vi "TicTacToe_pvp.vi"() -> ()   [LabVIEW 2020]
panel:
  in  "Turn 2":bool
  out "Human Win":dbl
  in  "Show XO plate":bool
  out "Computer Win":dbl
  out "Tie":bool
  out "No one Won":bool
  out "Game Over":bool
  out "Computer Won":bool
  out "Human Won":bool
  out "Turn":string
  out "XO array":string[][](array[string])
  in  "START GAME":bool
  in  "Boolean 9":bool
  in  "Boolean 8":bool
  in  "Boolean 7":bool
  in  "Boolean 6":bool
  in  "Boolean 5":bool
  in  "Boolean 4":bool
  in  "Boolean 3":bool
  in  "Boolean 2":bool
  in  "Boolean":bool
  in  "STOP GAME":bool
  in  "Turn":bool
  # "XO GAME"
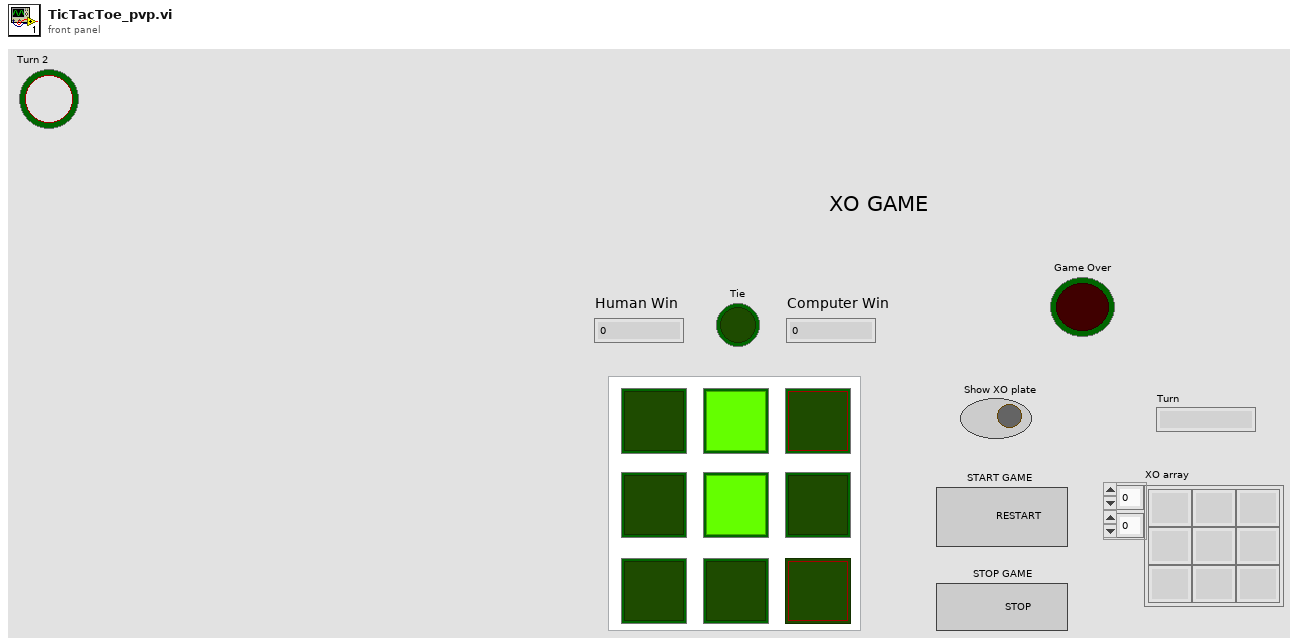
[diagram p1: front panel]
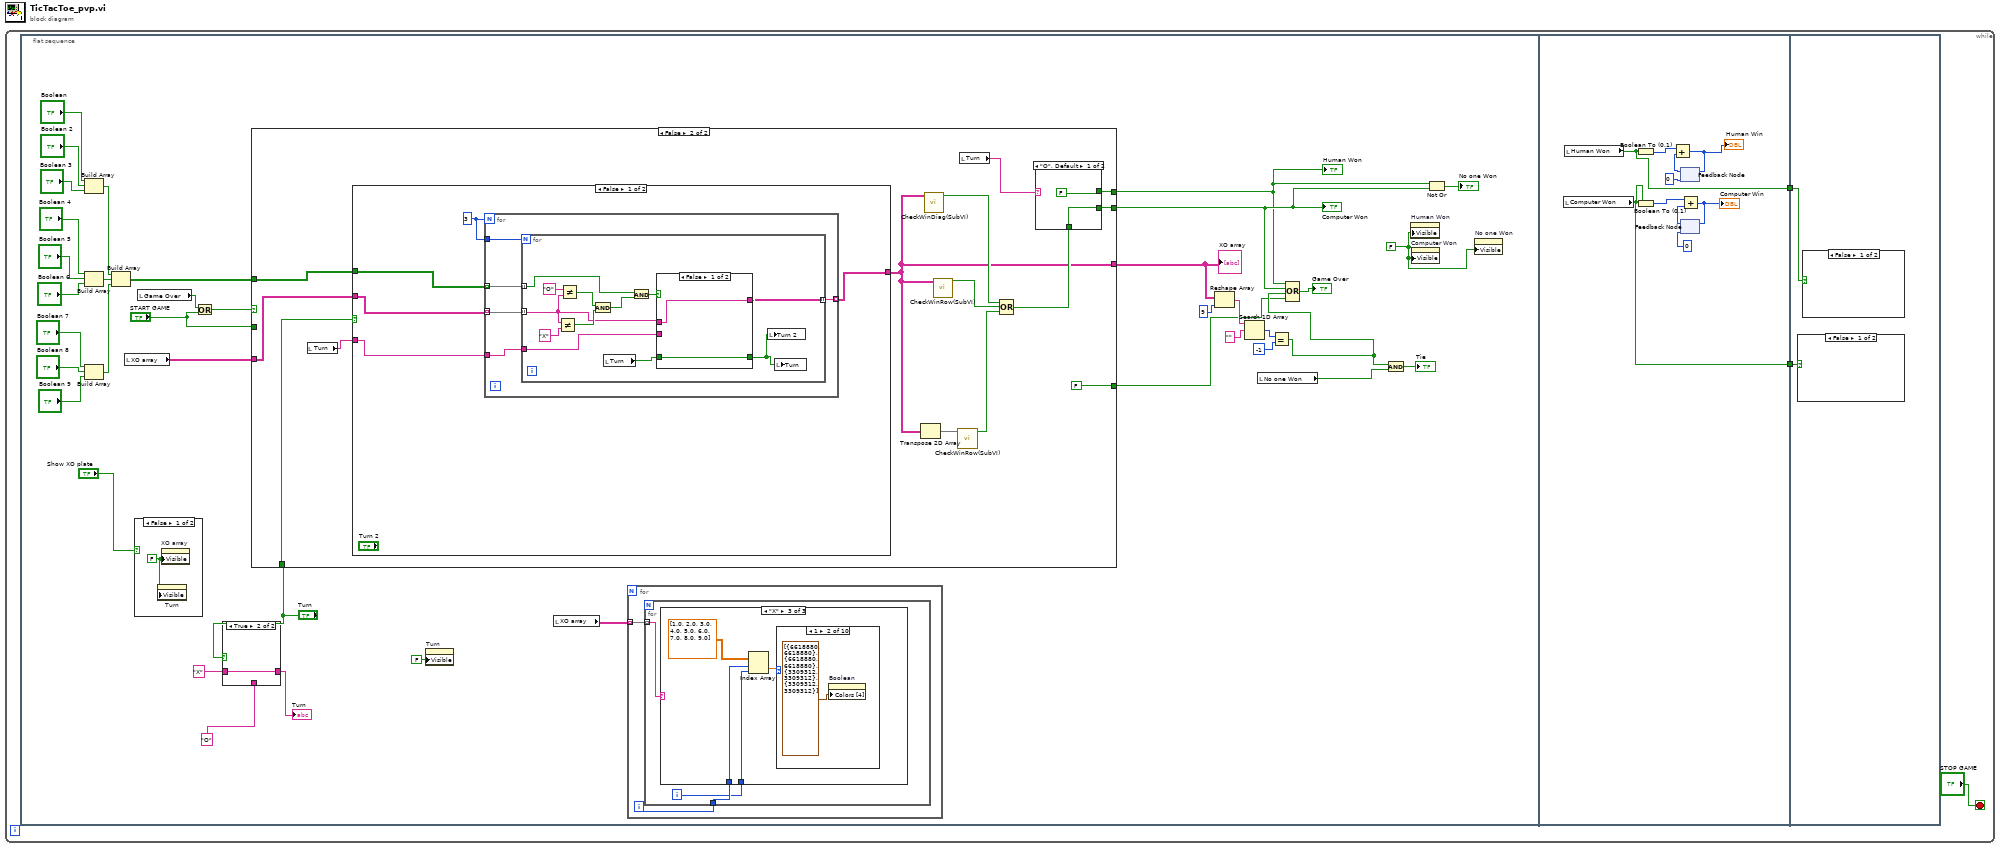
[diagram p0: block diagram]
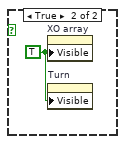
[diagram p2: hidden frame]
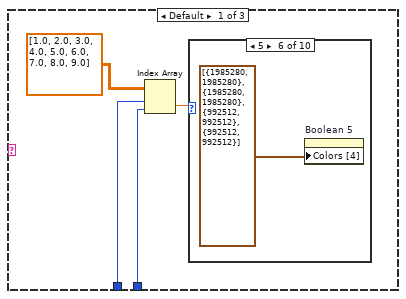
[diagram p3: hidden frame]
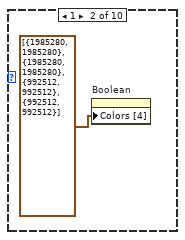
[diagram p5: hidden frame]
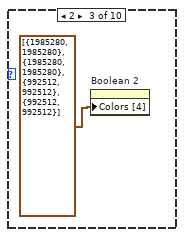
[diagram p6: hidden frame]
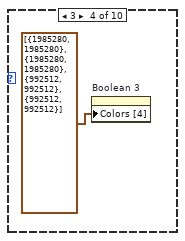
[diagram p7: hidden frame]
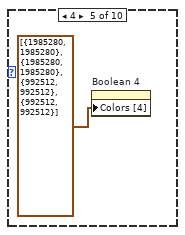
[diagram p8: hidden frame]
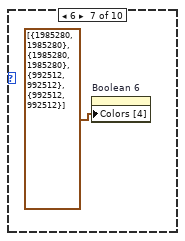
[diagram p9: hidden frame]
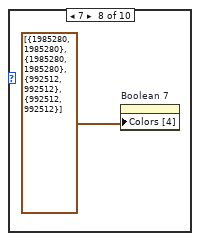
[diagram p10: hidden frame]
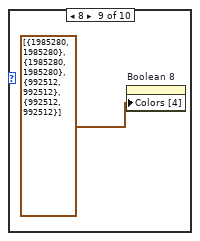
[diagram p11: hidden frame]
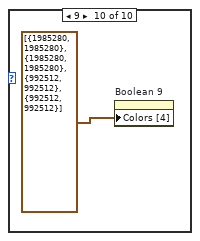
[diagram p12: hidden frame]
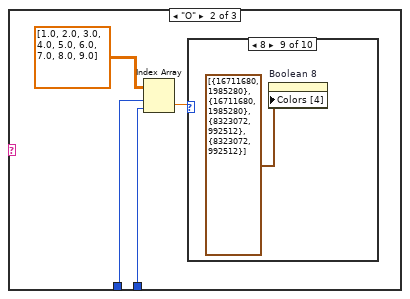
[diagram p13: hidden frame]
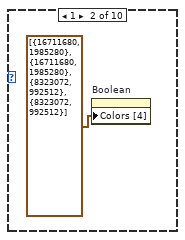
[diagram p15: hidden frame]
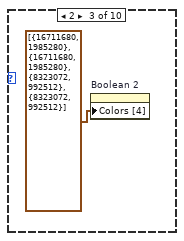
[diagram p16: hidden frame]
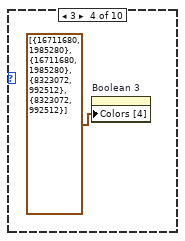
[diagram p17: hidden frame]
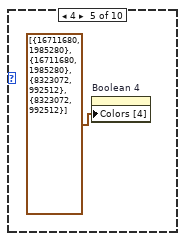
[diagram p18: hidden frame]
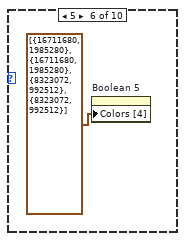
[diagram p19: hidden frame]
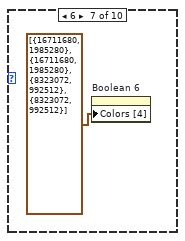
[diagram p20: hidden frame]
diagram:
  n1 = while {
    stop <- "STOP GAME" stop-if-true
    n2 = flat-sequence {
      tunnel: [w179] -> w2
      tunnel: [w178] -> w1
      tunnel: w2 -> [w189]
      tunnel: w1 -> [w188]
      frame #0 {
        w5 = FALSE ("Visible")
        n3 = Build Array("Boolean", "Boolean 2", "Boolean 3") -> (w40:bool[])
        n4 = Build Array("Boolean 4", "Boolean 5", "Boolean 6") -> (w41:bool[])
        n5 = Build Array("Boolean 7", "Boolean 8", "Boolean 9") -> (w42:bool[])
        n6 = Build Array(w40, w41, w42) -> (w32:bool[][])
        n7 = local read "XO array"() -> (w31:string[][])
        n8 = case shown="False" "Show XO plate" {
          frame False {
            w43 = FALSE ("Visible")
            n9 = property on="Turn" class="Str"("Visible"=w43) -> ()  [unwired: 2 in, 2 out]
            n10 = property on="XO array" class="Arr (strict)"("Visible"=w43) -> ()  [unwired: 2 in, 2 out]
          }
          frame True {
            w44 = TRUE ("Visible")
            n11 = property on="XO array" class="Arr (strict)"("Visible"=w44) -> ()  [unwired: 2 in, 2 out]
            n12 = property on="Turn" class="Str"("Visible"=w44) -> ()  [unwired: 2 in, 2 out]
          }
        }
        n13 = local read "Game Over"() -> (w24:bool)
        n14 = Or(x=w24, y="START GAME") -> (x .or. y?=w23:bool)
        n15 = case shown="True" "Turn" {
          tunnel: "X" -> [_ w90]
          tunnel: [w89 w90] -> w29
          tunnel: "O" ("x") -> [w89 _]
          frame False {
          }
          frame True {
          }
        }
        "Turn" <- w29
        n16 = case shown="False" w23 {
          tunnel: w32 -> [_ w119]
          tunnel: w31 -> [w95 w118]
          tunnel: "Turn" -> [_ w116]
          tunnel: "START GAME" -> [w96 _]
          tunnel: [w94 w109] -> w7
          tunnel: [w93 w108] -> w6
          tunnel: [w92 w107] -> w11
          tunnel: [w91 FALSE] -> w4
          frame True {
            n17 = case shown="True" w96 {
              tunnel: [w99 w104] -> w92
              tunnel: [w98 w103] -> w93
              tunnel: [w98 w103] -> w94
              tunnel: w95 -> [w99 _]
              tunnel: [TRUE FALSE] -> w91
              frame False {
                w98 = FALSE
              }
              frame True {
                w101 = FALSE
                w103 = FALSE
                w102 = 3
                n18 = local write "Boolean"(w101) -> ()
                n19 = local write "Boolean 2"(w101) -> ()
                n20 = local write "Boolean 3"(w101) -> ()
                n21 = local write "Boolean 6"(w101) -> ()
                n22 = local write "Boolean 5"(w101) -> ()
                n23 = local write "Boolean 7"(w101) -> ()
                n24 = local write "Boolean 8"(w101) -> ()
                n25 = local write "Boolean 9"(w101) -> ()
                n26 = local write "Boolean 4"(w101) -> ()
                n27 = Initialize Array("", w102, w102) -> (w104:string[][])
              }
            }
          }
          frame False {
            n28 = local read "Turn"() -> (w117:string)
            n29 = case shown="False" w116 {
              tunnel: w119 -> [w127 w155]
              tunnel: w118 -> [w126 w153]
              tunnel: [w124 w152] -> w107
              tunnel: w117 -> [w125 w151]
              frame False {
                w128 = 3
                n30 = for {
                  N: w128 -> [_]
                  tunnel: w128 -> [w133]
                  tunnel: w127 -> [w132] mode=indexing
                  tunnel: w126 -> [w131] mode=indexing
                  tunnel: [w130] -> w124 mode=indexing
                  tunnel: w125 -> [w129]
                  n31 = for {
                    N: w133 -> [_]
                    tunnel: w132 -> [w141] mode=indexing
                    tunnel: w131 -> [w138] mode=indexing
                    tunnel: w129 -> [w136]
                    tunnel: [w137] -> w130 mode=indexing
                    n32 = Not Equal?(x=w138, y="X") -> (x != y?=w142:bool)
                    n33 = Not Equal?(x="O", y=w138) -> (x != y?=w143:bool)
                    n34 = And(x=w143, y=w142) -> (x .and. y?=w140:bool)
                    n35 = local read "Turn"() -> (w135:bool)
                    n36 = And(x=w141, y=w140) -> (x .and. y?=w139:bool)
                    n37 = case shown="False" w139 {
                      tunnel: w138 -> [w147 _]
                      tunnel: [w147 w148] -> w137
                      tunnel: w136 -> [_ w148]
                      tunnel: [w146 w149] -> w134
                      tunnel: w135 -> [w146 w150]
                      frame False {
                      }
                      frame True {
                        n38 = Not(x=w150) -> (.not. x?=w149:bool)
                      }
                    }
                    n39 = local write "Turn 2"(w134) -> ()
                    n40 = local write "Turn"(w134) -> ()
                  }
                }
              }
              frame True {
                w154 = 3
                n41 = for {
                  N: w154 -> [_]
                  tunnel: w154 -> [w160]
                  tunnel: w155 -> [w159] mode=indexing
                  tunnel: w153 -> [w158] mode=indexing
                  tunnel: [w157] -> w152 mode=indexing
                  tunnel: w151 -> [w156]
                  n42 = for {
                    N: w160 -> [_]
                    tunnel: w159 -> [w168] mode=indexing
                    tunnel: w158 -> [w165] mode=indexing
                    tunnel: w156 -> [w163]
                    tunnel: [w164] -> w157 mode=indexing
                    n43 = Not Equal?(x=w165, y="X") -> (x != y?=w169:bool)
                    n44 = Not Equal?(x="O", y=w165) -> (x != y?=w170:bool)
                    n45 = And(x=w170, y=w169) -> (x .and. y?=w167:bool)
                    n46 = local read "Turn"() -> (w161:bool)
                    n47 = And(x=w168, y=w167) -> (x .and. y?=w166:bool)
                    n48 = case shown="True" w166 {
                      tunnel: w165 -> [w173 _]
                      tunnel: [w173 w175] -> w164
                      tunnel: w163 -> [_ w175]
                      tunnel: [w174 w176] -> w162
                      tunnel: w161 -> [w174 w177]
                      frame False {
                      }
                      frame True {
                        n49 = Not(x=w177) -> (.not. x?=w176:bool)
                      }
                    }
                    n50 = local write "Turn"(w162) -> ()
                  }
                }
              }
            }
            n51 = Transpose 2D Array(2D array=w107) -> (transposed array=w115:string[][])
            n52 = call "CheckWinDiag(SubVI).vi"("Array"=w107) -> ("x .or. y?"=w114:bool)  [unwired: 10 in]
            n53 = call "CheckWinRow(SubVI).vi"("Array"=w107) -> ("x .or. y? 2"=w113:bool)  [unwired: 10 in]
            n54 = call "CheckWinRow(SubVI).vi"("Array"=w115) -> ("x .or. y? 2"=w112:bool)  [unwired: 10 in]
            n55 = local read "Turn"() -> (w110:string)
            n56 = Compound Arithmetic op=OR(w114, w113, w112) -> (w111:bool)
            n57 = case shown="\"O\", Default" w110 {
              tunnel: w111 -> [w121 w122]
              tunnel: [w121 FALSE] -> w109
              tunnel: [FALSE w122] -> w108
              frame "O", Default {
              }
              frame "X" {
              }
            }
          }
        }
        "Human Won" <- w6
        "Computer Won" <- w7
        "XO array" <- w11
        n58 = property on="Turn" class="Bool (strict)"("Visible"=FALSE) -> ()  [unwired: 2 in, 2 out]
        n59 = local read "XO array"() -> (w10:string[][])
        n60 = for {
          tunnel: w10 -> [w45] mode=indexing
          i -> [w46]
          n61 = for {
            tunnel: w46 -> [w49]
            tunnel: w45 -> [w47] mode=indexing
            i -> [w48]
            n62 = case shown="\"X\"" w47 {
              tunnel: w49 -> [w53 w64 w77]
              tunnel: w48 -> [w52 w63 w78]
              frame Default {
                n63 = Index Array(array=dbl[][] [[1.0, 2.0, 3.0], [4.0, 5.0, 6.0], [7.0, 8.0, 9.0]] ("Array"), index (row)=w53, index (col)=w52) -> (element=w50:dbl)
                n64 = case shown="5" w50 {
                  frame 0, Default {
                  }
                  frame 1 {
                    n65 = property on="Boolean" class="Bool (strict)"("Colors [4]"=cluster{u32, u32}[] [{1985280, 1985280}, {1985280, 1985280}, {992512, 992512}, {992512, 992512}]) -> ()  [unwired: 2 in, 2 out]
                  }
                  frame 2 {
                    n66 = property on="Boolean 2" class="Bool (strict)"("Colors [4]"=cluster{u32, u32}[] [{1985280, 1985280}, {1985280, 1985280}, {992512, 992512}, {992512, 992512}]) -> ()  [unwired: 2 in, 2 out]
                  }
                  frame 3 {
                    n67 = property on="Boolean 3" class="Bool (strict)"("Colors [4]"=cluster{u32, u32}[] [{1985280, 1985280}, {1985280, 1985280}, {992512, 992512}, {992512, 992512}]) -> ()  [unwired: 2 in, 2 out]
                  }
                  frame 4 {
                    n68 = property on="Boolean 4" class="Bool (strict)"("Colors [4]"=cluster{u32, u32}[] [{1985280, 1985280}, {1985280, 1985280}, {992512, 992512}, {992512, 992512}]) -> ()  [unwired: 2 in, 2 out]
                  }
                  frame 5 {
                    n69 = property on="Boolean 5" class="Bool (strict)"("Colors [4]"=cluster{u32, u32}[] [{1985280, 1985280}, {1985280, 1985280}, {992512, 992512}, {992512, 992512}]) -> ()  [unwired: 2 in, 2 out]
                  }
                  frame 6 {
                    n70 = property on="Boolean 6" class="Bool (strict)"("Colors [4]"=cluster{u32, u32}[] [{1985280, 1985280}, {1985280, 1985280}, {992512, 992512}, {992512, 992512}]) -> ()  [unwired: 2 in, 2 out]
                  }
                  frame 7 {
                    n71 = property on="Boolean 7" class="Bool (strict)"("Colors [4]"=cluster{u32, u32}[] [{1985280, 1985280}, {1985280, 1985280}, {992512, 992512}, {992512, 992512}]) -> ()  [unwired: 2 in, 2 out]
                  }
                  frame 8 {
                    n72 = property on="Boolean 8" class="Bool (strict)"("Colors [4]"=cluster{u32, u32}[] [{1985280, 1985280}, {1985280, 1985280}, {992512, 992512}, {992512, 992512}]) -> ()  [unwired: 2 in, 2 out]
                  }
                  frame 9 {
                    n73 = property on="Boolean 9" class="Bool (strict)"("Colors [4]"=cluster{u32, u32}[] [{1985280, 1985280}, {1985280, 1985280}, {992512, 992512}, {992512, 992512}]) -> ()  [unwired: 2 in, 2 out]
                  }
                }
              }
              frame "O" {
                n74 = Index Array(array=dbl[][] [[1.0, 2.0, 3.0], [4.0, 5.0, 6.0], [7.0, 8.0, 9.0]] ("Array"), index (row)=w64, index (col)=w63) -> (element=w65:dbl)
                n75 = case shown="8" w65 {
                  frame 0, Default {
                  }
                  frame 1 {
                    n76 = property on="Boolean" class="Bool (strict)"("Colors [4]"=cluster{u32, u32}[] [{16711680, 1985280}, {16711680, 1985280}, {8323072, 992512}, {8323072, 992512}]) -> ()  [unwired: 2 in, 2 out]
                  }
                  frame 2 {
                    n77 = property on="Boolean 2" class="Bool (strict)"("Colors [4]"=cluster{u32, u32}[] [{16711680, 1985280}, {16711680, 1985280}, {8323072, 992512}, {8323072, 992512}]) -> ()  [unwired: 2 in, 2 out]
                  }
                  frame 3 {
                    n78 = property on="Boolean 3" class="Bool (strict)"("Colors [4]"=cluster{u32, u32}[] [{16711680, 1985280}, {16711680, 1985280}, {8323072, 992512}, {8323072, 992512}]) -> ()  [unwired: 2 in, 2 out]
                  }
                  frame 4 {
                    n79 = property on="Boolean 4" class="Bool (strict)"("Colors [4]"=cluster{u32, u32}[] [{16711680, 1985280}, {16711680, 1985280}, {8323072, 992512}, {8323072, 992512}]) -> ()  [unwired: 2 in, 2 out]
                  }
                  frame 5 {
                    n80 = property on="Boolean 5" class="Bool (strict)"("Colors [4]"=cluster{u32, u32}[] [{16711680, 1985280}, {16711680, 1985280}, {8323072, 992512}, {8323072, 992512}]) -> ()  [unwired: 2 in, 2 out]
                  }
                  frame 6 {
                    n81 = property on="Boolean 6" class="Bool (strict)"("Colors [4]"=cluster{u32, u32}[] [{16711680, 1985280}, {16711680, 1985280}, {8323072, 992512}, {8323072, 992512}]) -> ()  [unwired: 2 in, 2 out]
                  }
                  frame 7 {
                    n82 = property on="Boolean 7" class="Bool (strict)"("Colors [4]"=cluster{u32, u32}[] [{16711680, 1985280}, {16711680, 1985280}, {8323072, 992512}, {8323072, 992512}]) -> ()  [unwired: 2 in, 2 out]
                  }
                  frame 8 {
                    n83 = property on="Boolean 8" class="Bool (strict)"("Colors [4]"=cluster{u32, u32}[] [{16711680, 1985280}, {16711680, 1985280}, {8323072, 992512}, {8323072, 992512}]) -> ()  [unwired: 2 in, 2 out]
                  }
                  frame 9 {
                    n84 = property on="Boolean 9" class="Bool (strict)"("Colors [4]"=cluster{u32, u32}[] [{16711680, 1985280}, {16711680, 1985280}, {8323072, 992512}, {8323072, 992512}]) -> ()  [unwired: 2 in, 2 out]
                  }
                }
              }
              frame "X" {
                n85 = Index Array(array=dbl[][] [[1.0, 2.0, 3.0], [4.0, 5.0, 6.0], [7.0, 8.0, 9.0]] ("Array"), index (row)=w77, index (col)=w78) -> (element=w79:dbl)
                n86 = case shown="1" w79 {
                  frame 0, Default {
                  }
                  frame 1 {
                    n87 = property on="Boolean" class="Bool (strict)"("Colors [4]"=cluster{u32, u32}[] [{6618880, 6618880}, {6618880, 6618880}, {3309312, 3309312}, {3309312, 3309312}]) -> ()  [unwired: 2 in, 2 out]
                  }
                  frame 2 {
                    n88 = property on="Boolean 2" class="Bool (strict)"("Colors [4]"=cluster{u32, u32}[] [{6618880, 6618880}, {6618880, 6618880}, {3309312, 3309312}, {3309312, 3309312}]) -> ()  [unwired: 2 in, 2 out]
                  }
                  frame 3 {
                    n89 = property on="Boolean 3" class="Bool (strict)"("Colors [4]"=cluster{u32, u32}[] [{6618880, 6618880}, {6618880, 6618880}, {3309312, 3309312}, {3309312, 3309312}]) -> ()  [unwired: 2 in, 2 out]
                  }
                  frame 4 {
                    n90 = property on="Boolean 4" class="Bool (strict)"("Colors [4]"=cluster{u32, u32}[] [{6618880, 6618880}, {6618880, 6618880}, {3309312, 3309312}, {3309312, 3309312}]) -> ()  [unwired: 2 in, 2 out]
                  }
                  frame 5 {
                    n91 = property on="Boolean 5" class="Bool (strict)"("Colors [4]"=cluster{u32, u32}[] [{6618880, 6618880}, {6618880, 6618880}, {3309312, 3309312}, {3309312, 3309312}]) -> ()  [unwired: 2 in, 2 out]
                  }
                  frame 6 {
                    n92 = property on="Boolean 6" class="Bool (strict)"("Colors [4]"=cluster{u32, u32}[] [{6618880, 6618880}, {6618880, 6618880}, {3309312, 3309312}, {3309312, 3309312}]) -> ()  [unwired: 2 in, 2 out]
                  }
                  frame 7 {
                    n93 = property on="Boolean 7" class="Bool (strict)"("Colors [4]"=cluster{u32, u32}[] [{6618880, 6618880}, {6618880, 6618880}, {3309312, 3309312}, {3309312, 3309312}]) -> ()  [unwired: 2 in, 2 out]
                  }
                  frame 8 {
                    n94 = property on="Boolean 8" class="Bool (strict)"("Colors [4]"=cluster{u32, u32}[] [{6618880, 6618880}, {6618880, 6618880}, {3309312, 3309312}, {3309312, 3309312}]) -> ()  [unwired: 2 in, 2 out]
                  }
                  frame 9 {
                    n95 = property on="Boolean 9" class="Bool (strict)"("Colors [4]"=cluster{u32, u32}[] [{6618880, 6618880}, {6618880, 6618880}, {3309312, 3309312}, {3309312, 3309312}]) -> ()  [unwired: 2 in, 2 out]
                  }
                }
              }
            }
          }
        }
        n96 = Reshape Array(w11, 9 ("dimension size")) -> (w17:string[])
        n97 = Search 1D Array(1D array=w17, element="") -> (index of element=w15:i32)  [unwired: 1 in]
        n98 = local read "No one Won"() -> (w19:bool)
        n99 = Equal?(x=w15, y=-1) -> (x = y?=w12:bool)
        n100 = Compound Arithmetic op=OR(w6, w7, w12, w4) -> (→"Game Over":bool)
        n101 = And(x=w12, y=w19) -> (x .and. y?=→"Tie":bool)
        n102 = property on="Human Won" class="Bool (strict)"("Visible"=w5) -> ()  [unwired: 2 in, 2 out]
        n103 = property on="Computer Won" class="Bool (strict)"("Visible"=w5) -> ()  [unwired: 2 in, 2 out]
        n104 = Not Or(1:w7, 2:w6) -> (0:→"No one Won":bool)
        n105 = property on="No one Won" class="Bool (strict)"("Visible"=w5) -> ()  [unwired: 2 in, 2 out]
      }
      frame #1 {
        n106 = local read "Computer Won"() -> (w179:bool)
        n107 = local read "Human Won"() -> (w178:bool)
        n108 = Boolean To (0,1)(Boolean=w178) -> (0, 1=w182:i16)
        n109 = Boolean To (0,1)(Boolean=w179) -> (0, 1=w180:i16)
        n110 = feedback #1(i16 0) -> (w183:i16)
        n111 = Add(x=w182, y=w183) -> (x+y=w185:i16)
        "Human Win" <- w185
        n112 = feedback-in #1(w185) -> ()
        n113 = feedback #2(i16 0) -> (w181:i16)
        n114 = Add(x=w180, y=w181) -> (x+y=w184:i16)
        "Computer Win" <- w184
        n115 = feedback-in #2(w184) -> ()
      }
      frame #2 {
        n116 = case shown="False" w189 {
          frame False {
          }
          frame True {
            n117 = One Button Dialog(message="Computer Won") -> ()  [unwired: 1 in, 1 out]
          }
        }
        n118 = case shown="False" w188 {
          frame False {
          }
          frame True {
            n119 = One Button Dialog(message="Human WON") -> ()  [unwired: 1 in, 1 out]
          }
        }
      }
    }
  }
